vi "ControlSteerAngle.vi"(1 "Braking":bool, 2 "Robot Motion Commands":T1) -> (0 "output cluster":T1)   [LabVIEW 2018]
uses:
  Controls/Robot Pivot Motion Commands.ctl
  Controls/Pivot Motor Commands.ctl
  Controls/Robot Drive Mode.ctl
  <vilib>/Rock Robotics/WPI/Utilities/WPI_GetSetVariantRefNum.vi
  <vilib>/addons/control/pid/pid.llb/PID (DBL Array).vi
  <vilib>/addons/control/pid/NI_PID_pid.lvlib
panel:
  in  "Robot Motion Commands 2":T1
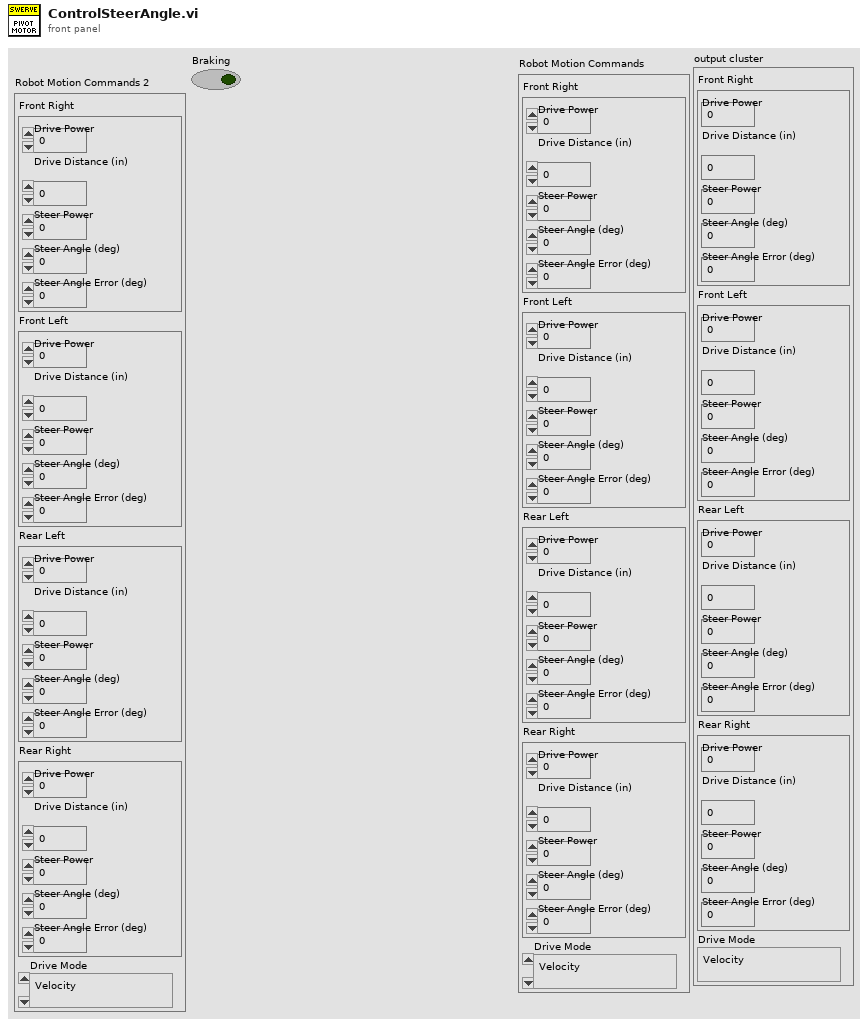
[diagram p1: front panel]
types:
  T1 = typedef "Robot Pivot Motion Commands.ctl" = cluster{"Front Right":T2, "Front Left":T2, "Rear Left":T2, "Rear Right":T2, "Drive Mode":T3}
  T2 = typedef "Pivot Motor Commands.ctl" = cluster{"Drive Power":dbl, "Drive Distance (in)":dbl, "Steer Power":dbl, "Steer Angle (deg)":dbl, "Steer Angle Error (deg)":dbl}
  T3 = typedef "Robot Drive Mode.ctl" = enum16{"Velocity", "Distance"}
  T4 = cluster{"proportional gain (Kc)":dbl, "integral time (Ti, min)":dbl, "derivative time (Td, min)":dbl}
  T5 = cluster{"proportional gain (Kc)":dbl, "integral time (Ti, min)":dbl, "derivative time (Td, min)":dbl}[]
  T6 = typedef "WPI_RobotDriveDevRef.ctl" = cluster{"DevStatus":errorcluster, "Motors[]":T7[], "Square Inputs":bool, "Max Output":dbl}
  T7 = typedef "WPI_MotorControlDeviceRef.ctl" = cluster{"DeviceStatus":errorcluster, "Type":T8, "PWM":cluster{"PWM Channel":T9, "DeadBand":T10}, "CAN":cluster{"Device Number":u8, "SetOutput VI Ref":variant, "GetOutput VI Ref":variant, "Enable VI Ref":variant, "Disable VI Ref":variant, "Data":variant}, "Invert":bool, "DIO PWM":cluster{"PWM \"Enable\" Channel":T9, "DIOChannel":T11, "PWM Rate":dbl}}
  T8 = typedef "WPI_MotorControlType.ctl" = enum16{"PWM", "CAN", "DIO PWM"}
  T9 = typedef "FPGA_DIOPWMChannel.ctl" = enum8{"PWM 0", "PWM 1", "PWM 2", "PWM 3", "PWM 4", "PWM 5", "PWM 6", "PWM 7", "PWM 8", "PWM 9", "PWM MXP 0", "PWM MXP 1", "PWM MXP 2", "PWM MXP 3", "PWM MXP 4", "PWM MXP 5", "PWM MXP 6", "PWM MXP 7", "PWM MXP 8", "PWM MXP 9", "Invalid"}
  T10 = typedef "WPI_PWMDeadband.ctl" = cluster{"Name":string, "maxPositivePwm":i32, "minPositivePwm":i32, "centerPwm":i32, "maxNegativePwm":i32, "minNegativePwm":i32, "angularRange":u16}
  T11 = typedef "FPGA_DIOChannel.ctl" = enum8{"DIO 0", "DIO 1", "DIO 2", "DIO 3", "DIO 4", "DIO 5", "DIO 6", "DIO 7", "DIO 8", "DIO 9", "DIO MXP 0", "DIO MXP 1", "DIO MXP 2", "DIO MXP 3", "DIO MXP 4", "DIO MXP 5", "DIO MXP 6", "DIO MXP 7", "DIO MXP 8", "DIO MXP 9", "DIO MXP 10", "DIO MXP 11", "DIO MXP 12", "DIO MXP 13", "DIO MXP 14", "DIO MXP 15", "SPI Port CS1", "SPI Port CS2", "SPI Port CS3", "SPI Port MISO", "SPI Port MOSI", "Invalid"}
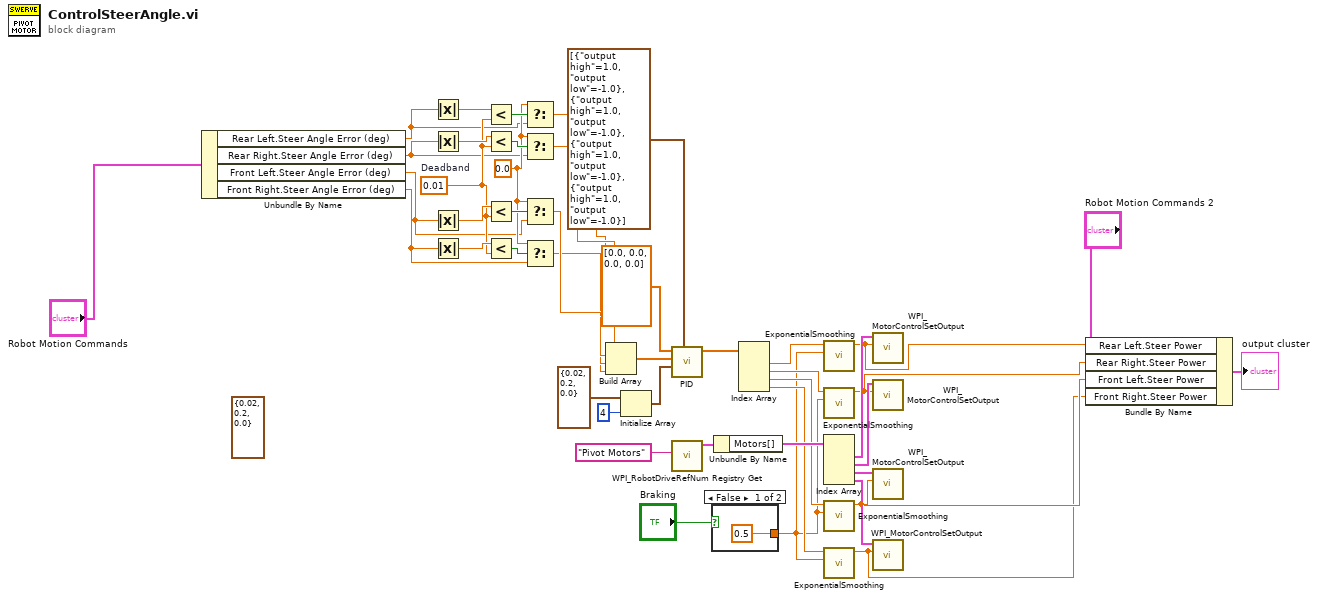
[diagram p0: block diagram]
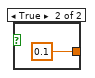
[diagram p2: hidden frame]
diagram:
  w10 = 0.0
  w5 = 0.01  # Deadband
  (unwired) T4 {"proportional gain (Kc)"=0.02, "integral time (Ti, min)"=0.2, "derivative time (Td, min)"=0.0} ("PID gains")
  n1 = Unbundle By Name("Robot Motion Commands") -> ("Rear Left.Steer Angle Error (deg)"=w4:dbl, "Rear Right.Steer Angle Error (deg)"=w3:dbl, "Front Left.Steer Angle Error (deg)"=w1:dbl, "Front Right.Steer Angle Error (deg)"=w2:dbl)
  n2 = Absolute Value(x=w4) -> (abs(x)=w12:dbl)
  n3 = Absolute Value(x=w3) -> (abs(x)=w14:dbl)
  n4 = Absolute Value(x=w1) -> (abs(x)=w16:dbl)
  n5 = Absolute Value(x=w2) -> (abs(x)=w18:dbl)
  n6 = Less?(x=w12, y=w5) -> (x < y?=w11:bool)
  n7 = Less?(x=w14, y=w5) -> (x < y?=w13:bool)
  n8 = Less?(x=w16, y=w5) -> (x < y?=w15:bool)
  n9 = Less?(x=w18, y=w5) -> (x < y?=w17:bool)
  n10 = Select(t=w10, s=w11, f=w4) -> (s? t:f=w9:dbl)
  n11 = Select(t=w10, s=w13, f=w3) -> (s? t:f=w8:dbl)
  n12 = Select(t=w10, s=w15, f=w1) -> (s? t:f=w7:dbl)
  n13 = Select(t=w10, s=w17, f=w2) -> (s? t:f=w6:dbl)
  n14 = Build Array(w9, w8, w7, w6) -> (w37:dbl[])
  n15 = Initialize Array(T4 {"proportional gain (Kc)"=0.02, "integral time (Ti, min)"=0.2, "derivative time (Td, min)"=0.0} ("PID gains"), 4 ("dimension size")) -> (w38:T5)
  n16 = call-poly <vilib>:"PID.vi"("output range"=cluster{"output high":dbl, "output low":dbl}[] [{"output high"=1.0, "output low"=-1.0}, {"output high"=1.0, "output low"=-1.0}, {"output high"=1.0, "output low"=-1.0}, {"output high"=1.0, "output low"=-1.0}], "PID gains"=w38, "process variable"=w37, "setpoint"=dbl[] [0.0, 0.0, 0.0, 0.0]) -> ("output"=w35:dbl[])  [unwired: 6 in, 1 out]
  n17 = call <vilib>:"WPI_RobotDriveRefNum Registry Get.vi"("refnum name"="Pivot Motors") -> ("RobotDriveDevRef"=w44:T6)  [unwired: 9 in, 1 out]
  n18 = case shown="False" "Braking" {
    tunnel: [0.5 ("Smoothing Factor") 0.1] -> w21
    frame False {
    }
    frame True {
    }
  }
  n19 = Unbundle By Name(w44) -> ("Motors[]"=w36:T7[])
  n20 = Index Array(array=w35) -> (element #1=w30:dbl, element #2=w29:dbl, element #3=w28:dbl, element #4=w27:dbl)  [unwired: 4 in]
  n21 = call "ExponentialSmoothing.vi"("Smoothing Factor"=w21, "Value"=w30) -> ("Smooth Value"=w22:dbl)  [unwired: 9 in]
  n22 = call "ExponentialSmoothing.vi"("Smoothing Factor"=w21, "Value"=w29) -> ("Smooth Value"=w26:dbl)  [unwired: 9 in]
  n23 = Index Array(array=w36) -> (element #1=w34:T7, element #2=w33:T7, element #3=w32:T7, element #4=w31:T7)  [unwired: 4 in]
  n24 = call "ExponentialSmoothing.vi"("Smoothing Factor"=w21, "Value"=w28) -> ("Smooth Value"=w25:dbl)  [unwired: 9 in]
  n25 = call "ExponentialSmoothing.vi"("Smoothing Factor"=w21, "Value"=w27) -> ("Smooth Value"=w24:dbl)  [unwired: 9 in]
  n26 = call <vilib>:"WPI_MotorControlSetOutput.vi"("Output"=w22, "MotorControlDevRef"=w34) -> ()  [unwired: 7 in, 3 out]
  n27 = call <vilib>:"WPI_MotorControlSetOutput.vi"("Output"=w26, "MotorControlDevRef"=w33) -> ()  [unwired: 7 in, 3 out]
  n28 = call <vilib>:"WPI_MotorControlSetOutput.vi"("Output"=w25, "MotorControlDevRef"=w32) -> ()  [unwired: 7 in, 3 out]
  n29 = call <vilib>:"WPI_MotorControlSetOutput.vi"("Output"=w24, "MotorControlDevRef"=w31) -> ()  [unwired: 7 in, 3 out]
  n30 = Bundle By Name(cluster="Robot Motion Commands 2", "Rear Left.Steer Power"=w22, "Rear Right.Steer Power"=w26, "Front Left.Steer Power"=w25, "Front Right.Steer Power"=w24) -> (→"output cluster":T1)
